vi "Parse 15-1.vi"(11 "String":string) -> (3 "Puzzle 15-1":T1)   [LabVIEW 2020]
uses:
  Puzzle 15-1.ctl
  Position.ctl
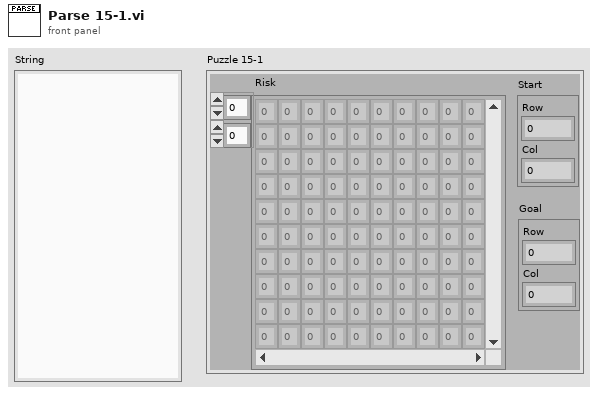
[diagram p1: front panel]
types:
  T1 = typedef "Puzzle 15-1.ctl" = cluster{"Risk":i32[][], "Start":T2, "Goal":T2}
  T2 = typedef "Position.ctl" = cluster{"Row":i32, "Col":i32}
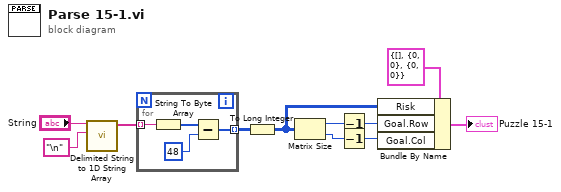
[diagram p0: block diagram]
diagram:
  n1 = call <vilib>:"Delimited String to 1D String Array.vi"("delimiter"="\n", "delimited string"="String") -> ("string array"=w9:string[])  [unwired: 9 in]
  n2 = for {
    tunnel: w9 -> [w15] mode=indexing
    tunnel: [w12] -> w8 mode=indexing
    n3 = String To Byte Array(string=w15) -> (unsigned byte array=w14:u8[])
    n4 = Subtract(x=w14, y=u8 48) -> (x-y=w12:u8[])
  }
  n5 = To Long Integer(number=w8) -> (32bit integer=w5:i32[][])
  n6 = Matrix Size(0:w5) -> (1:w2:i32, 2:w1:i32)
  n7 = Decrement(x=w2) -> (x-1=w4:i32)
  n8 = Decrement(x=w1) -> (x-1=w3:i32)
  n9 = Bundle By Name(cluster=T1 {"Risk"=[], "Start"={"Row"=0, "Col"=0}, "Goal"={"Row"=0, "Col"=0}} ("Puzzle 15-1"), "Risk"=w5, "Goal.Row"=w4, "Goal.Col"=w3) -> (→"Puzzle 15-1":T1)
